vi "U3 Read USB Descriptor Strings.vi"() -> (0 "error out":errorcluster)   [LabVIEW 2021]
panel:
  out "Data Array":u8[](array[numeric])
  out "iProduct":string
  out "iManufacturer":string
  in  "FirstFound":bool=TRUE
  in  "Address":string="1"
  out "Error Message":string
  # "Number of bytes in iManufacturer string"
  # "0x03"
  # "First character"
  # "0x00 (since Unicode)"
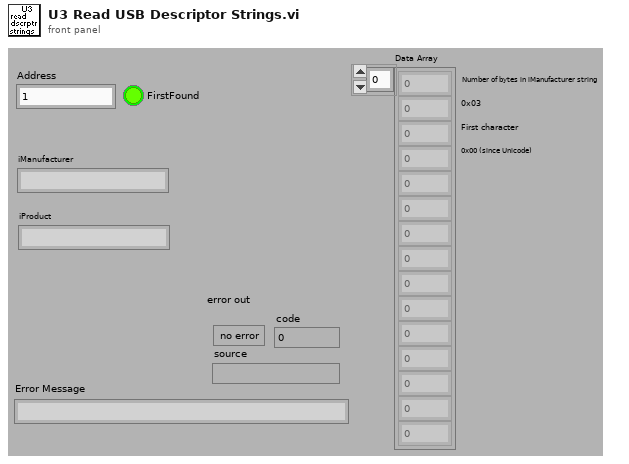
[diagram p1: front panel]
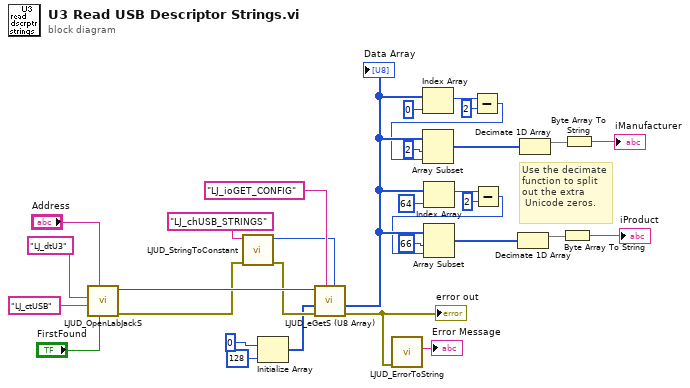
[diagram p0: block diagram]
diagram:
  # "Use the decimate\nfunction to split\nout the extra\n Unicode zeros."
  n1 = call "LJUD_OpenLabJackS.vi"("FirstFound"="FirstFound", "Address"="Address", "ConnectionType"="LJ_ctUSB", "DeviceType"="LJ_dtU3") -> ("error out"=w23:errorcluster, "Handle"=w26:i32)  [unwired: 5 in, 1 out]
  n2 = call "LJUD_StringToConstant.vi"("error in"=w23, "String"="LJ_chUSB_STRINGS" ("Channel")) -> ("error out"=w22:errorcluster, "Constant Number"=w21:i32)  [unwired: 8 in]
  n3 = Initialize Array(u8 0, 128 ("Dimension Size")) -> (w19:u8[])
  n4 = call "LJUD_eGetS (U8 Array).vi"("Channel"=w21, "IOType"="LJ_ioGET_CONFIG", "error in"=w22, "U8 Array Write"=w19, "Handle In"=w26) -> ("error out"=w29:errorcluster, "U8 Array Read"=w13:u8[])  [unwired: 3 in, 2 out]
  "error out" <- w29
  "Data Array" <- w13
  n5 = call "LJUD_ErrorToString.vi"("error in"=w29) -> ("String"=→"Error Message":string)  [unwired: 10 in]
  n6 = Index Array(array=w13, index=0 ("Index")) -> (element=w4:u8)
  n7 = Index Array(array=w13, index=64 ("Index")) -> (element=w2:u8)
  n8 = Subtract(x=w4, y=u8 2) -> (x-y=w3:u8)
  n9 = Array Subset(array=w13, index=2 ("Array Index"), length=w3) -> (w11:u8[])
  n10 = Subtract(x=w2, y=u8 2) -> (x-y=w1:u8)
  n11 = Array Subset(array=w13, index=66 ("Array Index"), length=w1) -> (w9:u8[])
  n12 = Decimate 1D Array(w9) -> (w10:u8[])  [unwired: 1 out]
  n13 = Decimate 1D Array(w11) -> (w7:u8[])  [unwired: 1 out]
  n14 = Byte Array To String(unsigned byte array=w10) -> (string=→"iProduct":string)
  n15 = Byte Array To String(unsigned byte array=w7) -> (string=→"iManufacturer":string)
